vi "Nested Loops.vi"() -> ()   [LabVIEW 2016]
panel:
  out "Loops":i32
  in  "stop":bool
  out "MOTOR":dbl(knob) scale=-1.0..1.0
  out "LAUNCH":bool
  in  "Launch":bool
  in  "Reverse":bool
  in  "Forward":bool
  # "Forward"
  # "Motor: -0.6"
  # "Launch: F"
  # "Reverse"
  # "Motor: 0.6"
  # "Launch: F"
  # "Launch"
  # "Motor: 0"
  # "Launch T"
  # "FORWARD"
  # "REVERSE"
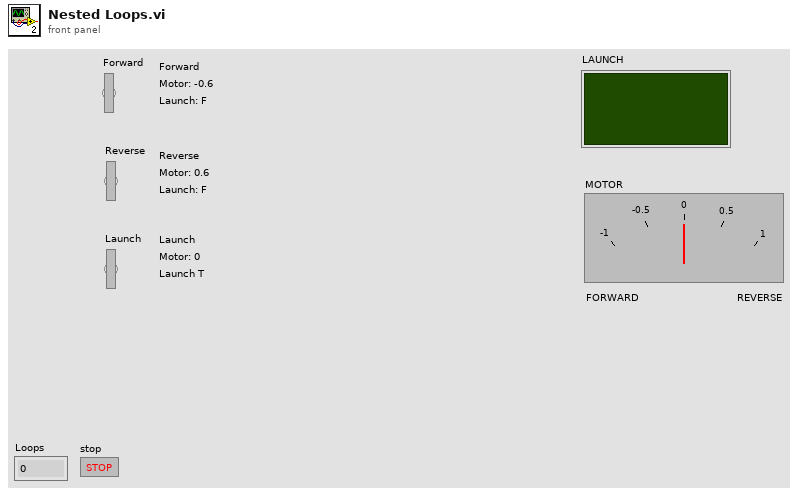
[diagram p1: front panel]
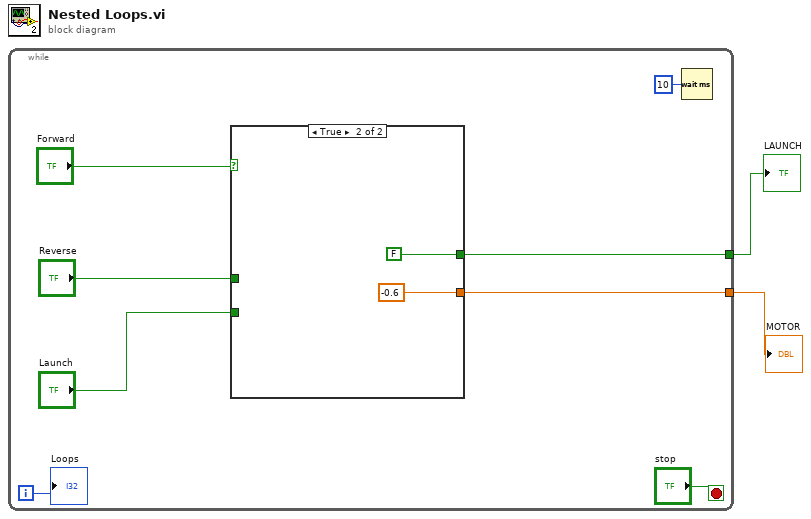
[diagram p0: block diagram]
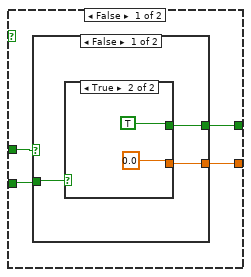
[diagram p2: hidden frame]
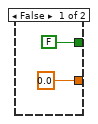
[diagram p3: hidden frame]
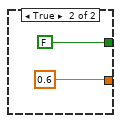
[diagram p4: hidden frame]
diagram:
  n1 = while {
    tunnel: [w4] -> w1
    tunnel: [w3] -> w2
    i -> [w5]
    stop <- "stop" stop-if-true
    n2 = case shown="True" "Forward" {
      tunnel: "Reverse" -> [w14 _]
      tunnel: "Launch" -> [w13 _]
      tunnel: [w12 FALSE ("LAUNCH")] -> w4
      tunnel: [w11 -0.6 ("MOTOR")] -> w3
      frame False {
        n3 = case shown="False" w14 {
          tunnel: w13 -> [w17 _]
          tunnel: [w16 FALSE ("LAUNCH")] -> w12
          tunnel: [w15 0.6 ("MOTOR")] -> w11
          frame False {
            n4 = case shown="True" w17 {
              tunnel: [FALSE ("LAUNCH") TRUE ("LAUNCH")] -> w16
              tunnel: [0.0 ("MOTOR") 0.0 ("MOTOR")] -> w15
              frame False {
              }
              frame True {
              }
            }
          }
          frame True {
          }
        }
      }
      frame True {
      }
    }
    n5 = Wait (ms)(milliseconds to wait=u32 10) -> ()  [unwired: 1 out]
    "Loops" <- w5
  }
  "LAUNCH" <- w1
  "MOTOR" <- w2
